vi "Read Arming (Trigger) Source.vi"(8 "error in (no error)":errorcluster, 11 "Pulse Generator in":refnum<class "Pulse Generator.lvclass">) -> (0 "error out":errorcluster, 2 "Arming (Trigger) Source":u16(ring)=2 items=["Immediate (Continuous Mode)", "Internal PLL", "External", "Manual"], 3 "Pulse Generator out":refnum<class "Pulse Generator.lvclass">)   [LabVIEW 2023, in "Pulse Generator.lvclass"]
uses:
  Pulse Generator.lvclass
  Pulse Generator.lvclass/Pulse Generator.ctl
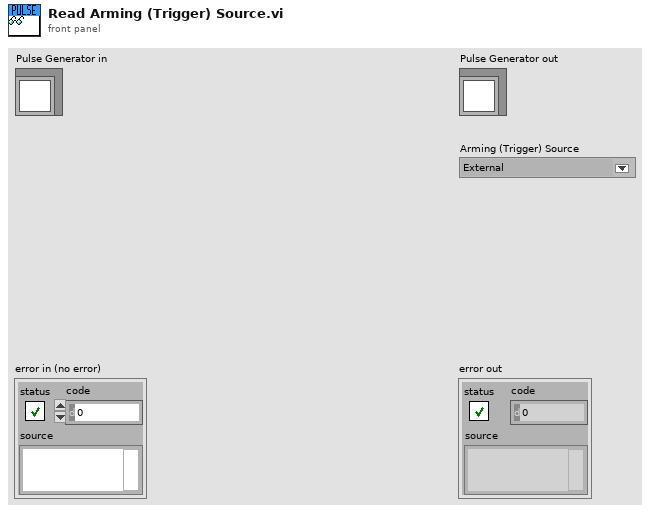
[diagram p1: front panel]
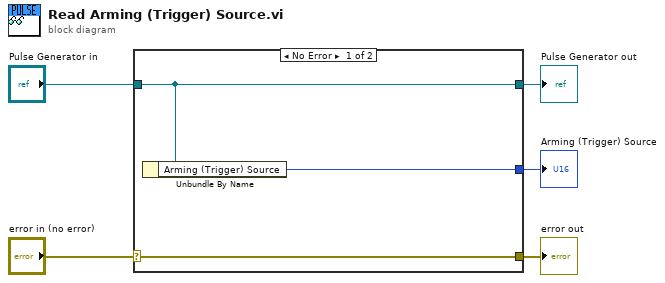
[diagram p0: block diagram]
diagram:
  n1 = case shown="No Error" "error in (no error)" {
    selector: "error in (no error)" -> [w8 w9]
    tunnel: [w8 w9] -> w4
    tunnel: [w7 w10] -> w2
    tunnel: "Pulse Generator in" -> [w7 w10]
    tunnel: [w6 _] -> w1
    frame No Error {
      n2 = Unbundle By Name(w7) -> ("Arming (Trigger) Source"=w6:u16)
    }
    frame Error {
    }
  }
  "error out" <- w4
  "Pulse Generator out" <- w2
  "Arming (Trigger) Source" <- w1
